vi "QRcodem.vi"() -> ()   [LabVIEW 2020]
uses:
  <vilib>/vision/Instrument.llb/QR Code Report.ctl
  <vilib>/vision/Instrument.llb/QR Code Model Type.ctl
  <vilib>/vision/Instrument.llb/QR Code Stream Mode Type.ctl
  <vilib>/vision/Instrument.llb/Data Matrix Polarity.ctl
  <vilib>/vision/Instrument.llb/Demodulation Mode.ctl
  <vilib>/vision/Instrument.llb/Cell Sample Size.ctl
  <vilib>/vision/Instrument.llb/Cell Filter Mode.ctl
panel:
  out "Array 2":bool[](array[boolean])
  out "Array":string[][](array[string])
  in  "ROT":dbl
  out "QR Barcode Report (2D Barcode Reader 1)":T1={"Found?"=FALSE, "Data"="", "Bounding Box"=[], "Errors Corrected"=0, "Dimensions (Rows/Cols)"=0, "Version"=0, "QR Model"=3, "Stream Mode"=0, "Barcode Polarity"=-2, "Mirrored?"=FALSE, "Append Stream Position"=0, "Size of Append Stream"=0, "First EAN-128 ID"=0, "First Alternate Language ID"=0, "Append Stream ID"=0, "Minimum Edge Strength"=30, "Demodulation Mode"=-2, "Cell Sample Size"=-2, "Cell Filter Mode"=-2} {"Append Stream ID" format="%x"; "Cell Filter Mode" items=["Auto-detect"=-2, "Average"=0, "Median"=1, "Central Average"=2, "High Average"=3, "Low Average"=4, "Very High Average"=5, "Very Low Average"=6, "All Filters"=8]; "Cell Sample Size" items=["Auto-detect"=-2, "1x1"=1, "2x2"=2, "3x3"=3, "4x4"=4, "5x5"=5, "6x6"=6, "7x7"=7]; "Demodulation Mode" items=["Auto-detect"=-2, "Histogram"=0, "Local Contrast"=1, "Combination"=2, "All"=3]; "Barcode Polarity" items=["Auto-detect"=-2, "Black on White"=0, "White on Black"=1]; "Stream Mode" items=["Auto-detect", "Numeric", "AlphaNumeric", "Mixed", "Raw Bytes", "UCC/EAN-128 - In Tokens", "UCC/EAN-128 - In Data", "Extended Character Interpretation", "Kanji"]; "QR Model" items=["Auto Detect", "Micro", "Model 1", "Model 2"]; "Version" max=40 step=1}
  in  "Stop (F)":bool
  out "Image Out":T8(plugin-control)
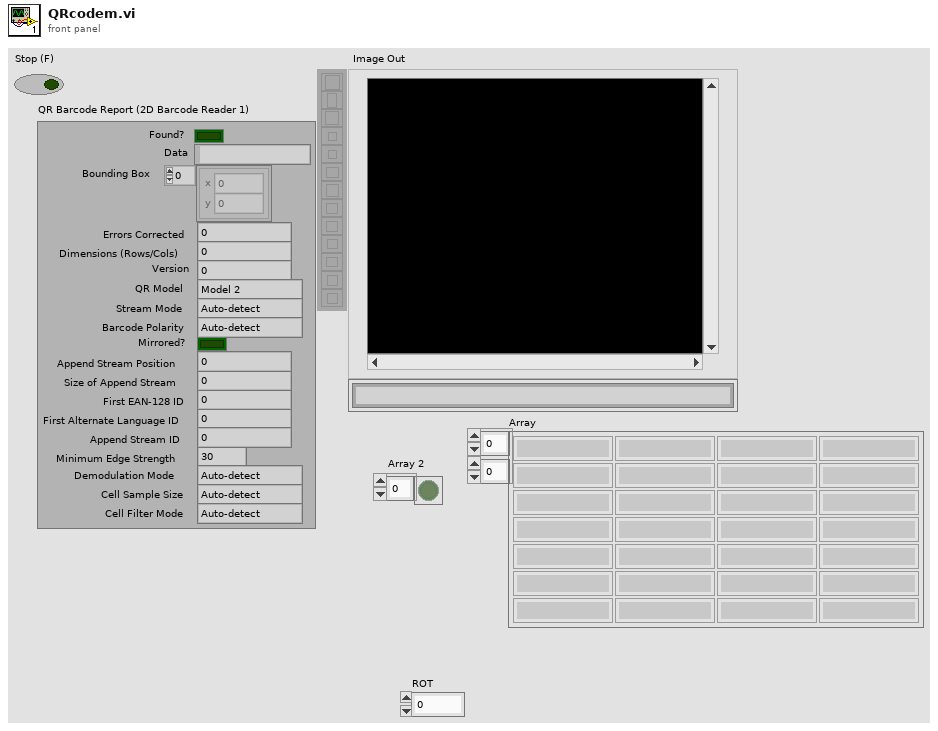
[diagram p1: front panel]
types:
  T1 = typedef "QR Code Report.ctl" = cluster{"Found?":bool, "Data":string, "Bounding Box":cluster{"x":sgl, "y":sgl}[], "Errors Corrected":u32, "Dimensions (Rows/Cols)":u32, "Version":u32, "QR Model":T2, "Stream Mode":T3, "Barcode Polarity":T4, "Mirrored?":bool, "Append Stream Position":u32, "Size of Append Stream":u32, "First EAN-128 ID":i32, "First Alternate Language ID":i32, "Append Stream ID":u32, "Minimum Edge Strength":u32, "Demodulation Mode":T5, "Cell Sample Size":T6, "Cell Filter Mode":T7}
  T2 = typedef "QR Code Model Type.ctl" = i32
  T3 = typedef "QR Code Stream Mode Type.ctl" = i32
  T4 = typedef "Data Matrix Polarity.ctl" = i32
  T5 = typedef "Demodulation Mode.ctl" = i32
  T6 = typedef "Cell Sample Size.ctl" = i32
  T7 = typedef "Cell Filter Mode.ctl" = i32
  T8 = typedef "IMAQ Image.ctl" = refnum<image>
  T9 = typedef "ROI Descriptor" = cluster{"Global Rectangle":i32[], "Contours":cluster{"ID":enum32{"External", "Internal"}, "Type":u32, "Coordinates":i32[]}[]}
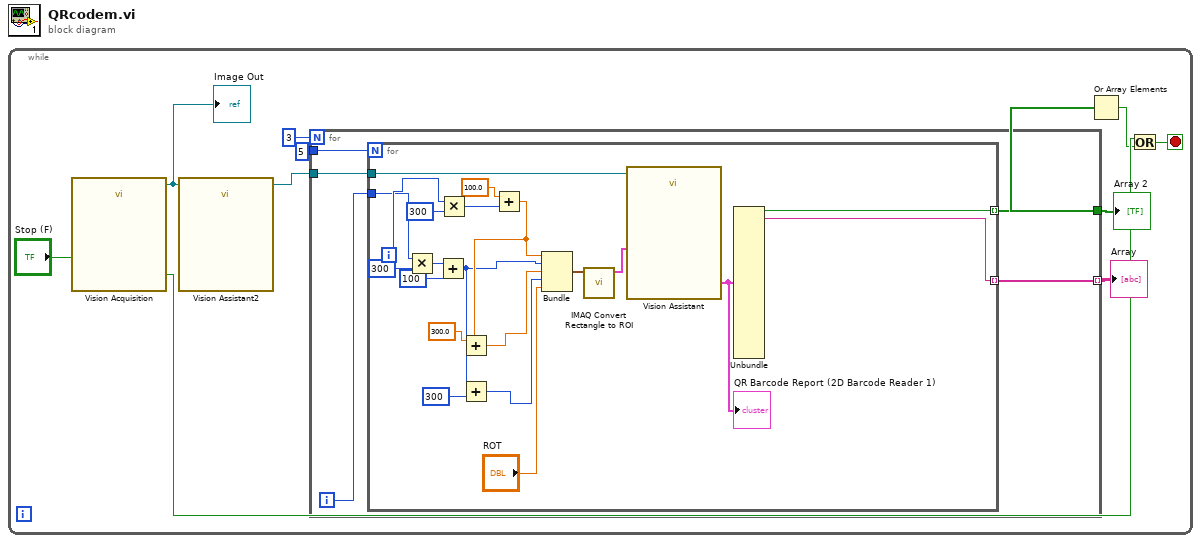
[diagram p0: block diagram]
diagram:
  n1 = while {
    stop <- w3 stop-if-true
    n2 = call "Vision Acquisition"("Stop (F)"="Stop (F)") -> ("Image Out"=w7:T8, "Stopped"=w4:bool)  [unwired: 24 in, 1 out]
    "Image Out" <- w7
    n3 = call "Vision Assistant2"("Image In"=w7) -> ("Image Out"=w6:T8)  [unwired: 25 in, 1 out]
    n4 = for {
      N: 3 -> [_]
      tunnel: 5 -> [w15]
      tunnel: [w14] -> w8 mode=indexing
      tunnel: w6 -> [w13]
      tunnel: [w12] -> w5
      i -> [w11]
      n5 = for {
        N: w15 -> [_]
        tunnel: w13 -> [w35]
        tunnel: [w33] -> w14 mode=indexing
        tunnel: [w27] -> w12 mode=indexing
        tunnel: w11 -> [w16]
        i -> [w17]
        n6 = Multiply(x=w16, y=300) -> (x*y=w22:i32)
        n7 = Add(x=w22, y=100) -> (x+y=w20:i32)
        n8 = Multiply(x=w17, y=300) -> (x*y=w32:i32)
        n9 = Add(x=w20, y=300) -> (x+y=w18:i32)
        n10 = Add(x=100.0, y=w32) -> (x+y=w24:dbl)
        n11 = Add(x=300.0, y=w24) -> (x+y=w25:dbl)
        n12 = Bundle(w24, w20, w25, w18, "ROT"="ROT") -> (w29:cluster{dbl, i32, dbl, i32, "ROT":dbl})  [unwired: 1 in]
        n13 = call "IMAQ Convert Rectangle to ROI"("Rectangle"=w29) -> ("ROI Descriptor"=w28:T9)  [unwired: 8 in, 1 out]
        n14 = call "Vision Assistant"("Image In"=w35, "ROI Descriptor (2D Barcode Reader 1)"=w28) -> ("QR Barcode Report (2D Barcode Reader 1)"=w34:T1)  [unwired: 23 in, 2 out]
        "QR Barcode Report (2D Barcode Reader 1)" <- w34
        n15 = Unbundle(w34) -> ("Found?"=w27:bool, "Data"=w33:string)  [unwired: 17 out]
      }
    }
    "Array" <- w8
    "Array 2" <- w5
    n16 = Or Array Elements(Boolean array=w5) -> (logical OR=w2:bool)
    n17 = Or(x=w4, y=w2) -> (x .or. y?=w3:bool)
  }
